vi "p3_Control_temperatura.vi"() -> ()   [LabVIEW 2019]
uses:
  Control_temp.ctl
panel:
  out "Decremento":bool
  out "Incremento":bool
  in  "Temp\nMin":sgl=25.0 min=0 max=200 step=1
  in  "Temp\nMax":sgl=150.0 min=0 max=200 step=1
  in  "Selector":bool
  in  "Decremento T":T1=1.0 scale=0.0..10.0
  in  "Incremento T":T1=1.0 scale=0.0..10.0
  in  "Rata de T(°C/seg)":T1=1.0 scale=1.0..10.0
  out "Sensor de Temperatura":dbl(slide) scale=0.0..200.0
  # "Decrementar"
  # "Incrementar"
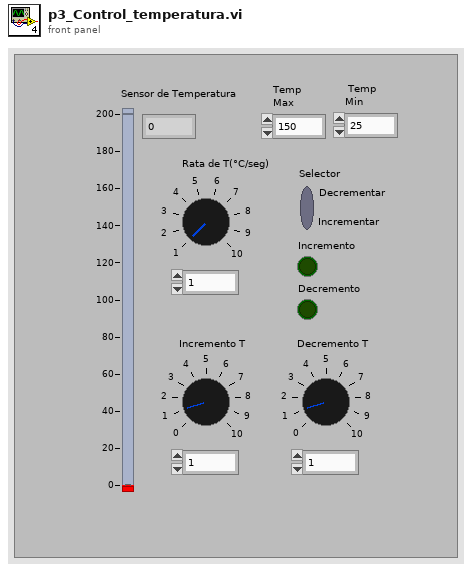
[diagram p1: front panel]
types:
  T1 = typedef "Control_temp.ctl" = dbl
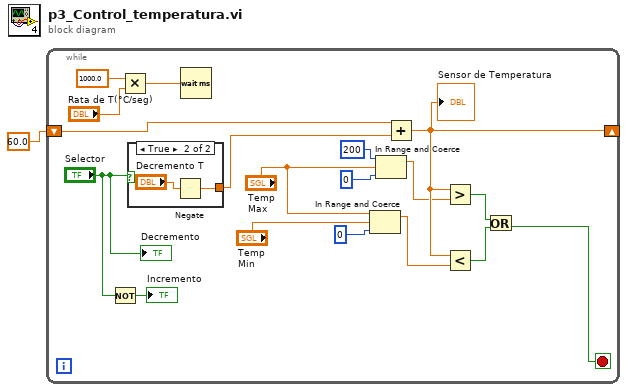
[diagram p0: block diagram]
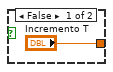
[diagram p2: hidden frame]
diagram:
  n1 = while {
    shift-right: [w13] -> _
    shift-left: T1 60.0 ("Decremento T") -> [w16]
    stop <- w10 stop-if-true
    n2 = Not(x="Selector") -> (.not. x?=→"Incremento":bool)
    n3 = Multiply(x=1000.0, y="Rata de T(°C/seg)") -> (x*y=w17:T1)
    n4 = case shown="True" "Selector" {
      tunnel: ["Incremento T" w21] -> w9
      frame False {
      }
      frame True {
        n5 = Negate(x="Decremento T") -> (-x=w21:T1)
      }
    }
    n6 = Wait (ms)(milliseconds to wait=w17) -> ()  [unwired: 1 out]
    n7 = In Range and Coerce(upper limit="Temp\nMax", x="Temp\nMin", lower limit=u8 0) -> (coerced(x)=w4:sgl)  [unwired: 1 out]
    n8 = In Range and Coerce(upper limit=u8 200, x="Temp\nMax", lower limit=u8 0) -> (coerced(x)=w6:sgl)  [unwired: 1 out]
    n9 = Add(x=w16, y=w9) -> (x+y=w13:T1)
    "Sensor de Temperatura" <- w13
    n10 = Greater?(x=w13, y=w6) -> (0:w12:bool)
    n11 = Less?(x=w13, y=w4) -> (x < y?=w11:bool)
    n12 = Or(x=w12, y=w11) -> (x .or. y?=w10:bool)
    "Decremento" <- "Selector"
  }
